vi "报警.vi"(8 "temp":string[](array[string]), 11 "fengshan":string[](array[string])) -> (2 "ALARM":bool)   [LabVIEW 2015]
panel:
  out "温度":string
  out "风扇":string
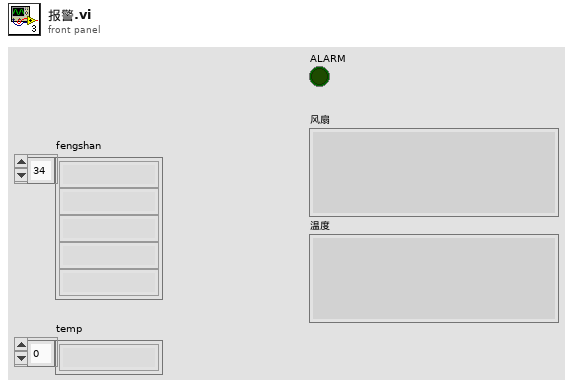
[diagram p1: front panel]
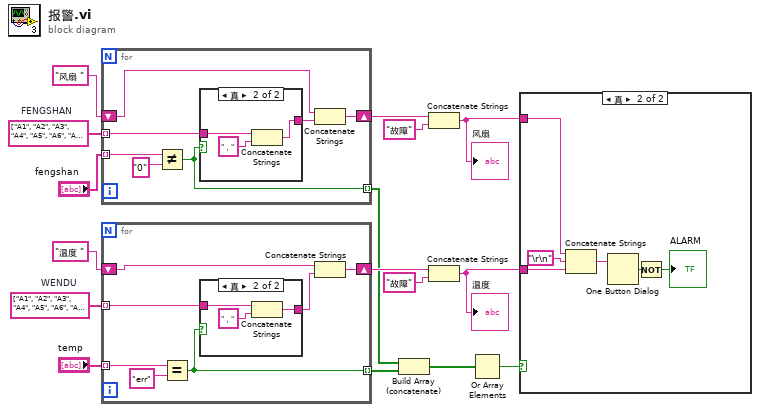
[diagram p0: block diagram]
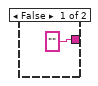
[diagram p3: hidden frame]
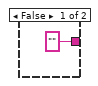
[diagram p4: hidden frame]
diagram:
  w15 = string[] ["A1", "A2", "A3", "A4", "A5", "A6", "A7", "A8", "A9", "A10", "A11", "A12", "A13", "A14", "A15", "A16", "A17", "A18", "A19", "A20", "A21", "A22", "A23", "A24", "A25", "A26", "A27", "A28", "A29", "A30", "A31", "A32", "主控A33", "主控A34", "主控A35", "主控A36", "B1", "B2", "B3", "B4", "B5", "B6", "B7", "B8", "B9", "B10", "B11", "B12", "B13", "B14", "B15", "B16", "B17", "B18", "B19", "B20", "B21", "B22", "B23", "B24", "B25", "B26", "B27", "B28", "B29", "B30", "B31", "B32", "主控B33", "主控B34", "主控B35", "主控B36"]  # FENGSHAN
  w10 = string[] ["A1", "A2", "A3", "A4", "A5", "A6", "A7", "A8", "A9", "A10", "A11", "A12", "A13", "A14", "A15", "A16", "A17", "A18", "A19", "A20", "A21", "A22", "A23", "A24", "A25", "A26", "A27", "A28", "A29", "A30", "A31", "A32", "A33", "A34", "A35", "A36", "A37", "A38", "A39", "A40", "A41", "A42", "A43", "A44", "A45", "A46", "A47", "A48", "A49", "A50", "A51", "A52", "A53", "A54", "A55", "A56", "A57", "A58", "A59", "A60", "A61", "A62", "A63", "A64", "主控A65", "主控A66", "B1", "B2", "B3", "B4", "B5", "B6", "B7", "B8", "B9", "B10", "B11", "B12", "B13", "B14", "B15", "B16", "B17", "B18", "B19", "B20", "B21", "B22", "B23", "B24", "B25", "B26", "B27", "B28", "B29", "B30", "B31", "B32", "B33", "B34", "B35", "B36", "B37", "B38", "B39", "B40", "B41", "B42", "B43", "B44", "B45", "B46", "B47", "B48", "B49", "B50", "B51", "B52", "B53", "B54", "B55", "B56", "B57", "B58", "B59", "B60", "B61", "B62", "B63", "B64", "主控B65", "主控B66"]  # WENDU
  n1 = for {
    tunnel: "fengshan" -> [w23] mode=indexing
    tunnel: w15 -> [w20] mode=indexing
    shift-right: [w21] -> w13
    shift-left: "风扇 " -> [w18]
    tunnel: [w17] -> w6 mode=indexing
    n2 = Not Equal?(x=w23, y="0") -> (x != y?=w17:bool)
    n3 = case shown="真" w17 {
      tunnel: w20 -> [_ w27]
      tunnel: ["" w25] -> w19
      frame False {
      }
      frame True {
        n4 = Concatenate Strings(w27, "，" ("string")) -> (w25:string)
      }
    }
    n5 = Concatenate Strings(w18, w19) -> (w21:string)
  }
  n6 = for {
    tunnel: "temp" -> [w34] mode=indexing
    tunnel: w10 -> [w30] mode=indexing
    shift-right: [w29] -> w7
    shift-left: "温度 " -> [w32]
    tunnel: [w28] -> w5 mode=indexing
    n7 = Equal?(x=w34, y="err") -> (x = y?=w28:bool)
    n8 = case shown="真" w28 {
      tunnel: ["" w37] -> w31
      tunnel: w30 -> [_ w36]
      frame False {
      }
      frame True {
        n9 = Concatenate Strings(w36, "，" ("string")) -> (w37:string)
      }
    }
    n10 = Concatenate Strings(w32, w31) -> (w29:string)
  }
  n11 = Build Array (concatenate)(w6, w5) -> (w4:bool[])
  n12 = Concatenate Strings(w13, "故障" ("string")) -> (w2:string)
  "风扇" <- w2
  n13 = Concatenate Strings(w7, "故障" ("string")) -> (w1:string)
  "温度" <- w1
  n14 = Or Array Elements(Boolean array=w4) -> (logical OR=w3:bool)
  n15 = case shown="真" w3 {
    tunnel: w2 -> [_ w43]
    tunnel: w1 -> [_ w42]
    frame False {
    }
    frame True {
      n16 = Concatenate Strings(w43, "\r\n", w42) -> (w41:string)
      n17 = One Button Dialog(message=w41) -> (true=w40:bool)  [unwired: 1 in]
      n18 = Not(x=w40) -> (.not. x?=→"ALARM":bool)
    }
  }
